vi "Handle.vi"(8 "error in (no error)":errorcluster, 11 "TelFocus in":refnum<class "TelFocus.lvclass">) -> (0 "error out":errorcluster, 3 "TelFocus out":refnum<class "TelFocus.lvclass">)   [LabVIEW 2018, in "TelFocus.lvclass"]
uses:
  TelFocus.lvclass
  TelFocus.lvclass/TelFocus.ctl
  Device/Device.lvclass/Device.ctl
  SecMirror/SecMirror.lvclass
  C:/Users/observer/Desktop/Sparc4GUI/Versao ZeroMQ/SPARC4_GUI -20240711_20240708/Device/Device.lvclass
  Server/Server.lvclass
  Comm/Stream/Stream.lvclass
  Device/Device.lvclass
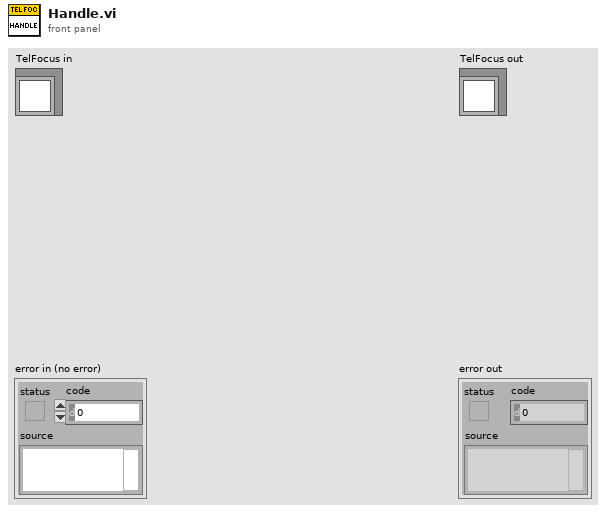
[diagram p1: front panel]
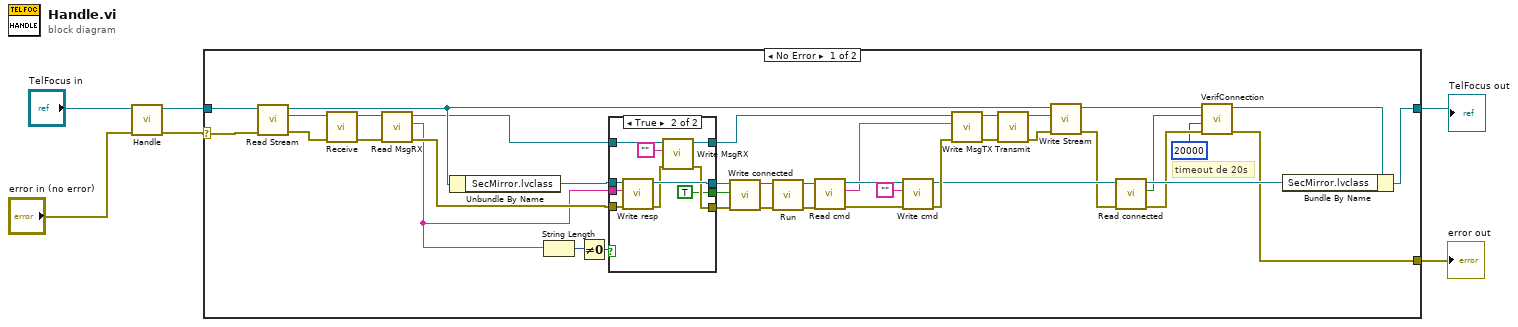
[diagram p0: block diagram]
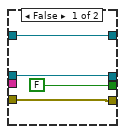
[diagram p2: hidden frame]
diagram:
  n1 = call-parent "Handle.vi"("error in (no error)"="error in (no error)", "Server in"="TelFocus in") -> ("error out"=w3:errorcluster, "Server out"=w4:refnum<class "TelFocus.lvclass">)  [unwired: 8 in]
  n2 = case shown="No Error" w3 {
    selector: w3 -> [w44 w62]
    tunnel: [w18 w62] -> w1
    tunnel: [w43 w61] -> w2
    tunnel: w4 -> [w35 w61]
    frame No Error {
      # "timeout de 20s"
      n3 = call-dynamic "Read Stream.vi"("error in (no error)"=w44, "Server in"=w35) -> ("error out"=w45:errorcluster, "Stream.lvclass"=w46:refnum<class "Stream.lvclass">, "Server out"=w37:refnum<class "TelFocus.lvclass">)  [unwired: 7 in]
      n4 = call-dynamic "Receive.vi"("error in (no error)"=w45, "Stream in"=w46) -> ("error out"=w42:errorcluster, "Stream out"=w41:refnum<class "Stream.lvclass">)  [unwired: 8 in]
      n5 = call-dynamic "Read MsgRX.vi"("error in (no error)"=w42, "Comm in"=w41) -> ("error out"=w15:errorcluster, "MsgRX"=w14:string, "Comm out"=w13:refnum<class "Stream.lvclass">)  [unwired: 7 in]
      n6 = Unbundle By Name(w37) -> ("SecMirror.lvclass"=w16:refnum<class "SecMirror.lvclass">)
      n7 = String Length(string=w14) -> (length=w29:i32)
      n8 = Not Equal To 0?(x=w29) -> (x != 0?=w28:bool)
      n9 = case shown="True" w28 {
        tunnel: [w49 w53] -> w9
        tunnel: [w50 w59] -> w10
        tunnel: w15 -> [w49 w58]
        tunnel: w16 -> [w50 w60]
        tunnel: w14 -> [_ w57]
        tunnel: w13 -> [w48 w56]
        tunnel: [w48 w55] -> w12
        tunnel: [FALSE TRUE] -> w11
        frame False {
        }
        frame True {
          n10 = call-dynamic "Write resp.vi"("error in (no error)"=w58, "resp"=w57, "Device in"=w60) -> ("error out"=w54:errorcluster, "Device out"=w59:refnum<class "SecMirror.lvclass">)  [unwired: 7 in]
          n11 = call-dynamic "Write MsgRX.vi"("error in (no error)"=w54, "MsgRX"="", "Comm in"=w56) -> ("error out"=w53:errorcluster, "Comm out"=w55:refnum<class "Stream.lvclass">)  [unwired: 7 in]
        }
      }
      n12 = call "Write connected.vi"("error in (no error)"=w9, "connected"=w11, "Device in"=w10) -> ("error out"=w7:errorcluster, "Device out"=w8:refnum<class "SecMirror.lvclass">)  [unwired: 7 in]
      n13 = call-dynamic "Run.vi"("error in (no error)"=w7, "SecMirror in"=w8) -> ("error out"=w26:errorcluster, "SecMirror out"=w27:refnum<class "SecMirror.lvclass">)  [unwired: 8 in]
      n14 = call-dynamic "Read cmd.vi"("error in (no error)"=w26, "Device in"=w27) -> ("error out"=w33:errorcluster, "cmd"=w31:string, "Device out"=w34:refnum<class "SecMirror.lvclass">)  [unwired: 7 in]
      n15 = call-dynamic "Write cmd.vi"("error in (no error)"=w33, "cmd"="", "Device in"=w34) -> ("error out"=w40:errorcluster, "Device out"=w25:refnum<class "SecMirror.lvclass">)  [unwired: 7 in]
      n16 = call-dynamic "Write MsgTX.vi"("error in (no error)"=w40, "MsgTX"=w31, "Comm in"=w12) -> ("error out"=w38:errorcluster, "Comm out"=w39:refnum<class "Stream.lvclass">)  [unwired: 7 in]
      n17 = call-dynamic "Transmit.vi"("error in (no error)"=w38, "Stream in"=w39) -> ("error out"=w36:errorcluster, "Stream out"=w30:refnum<class "Stream.lvclass">)  [unwired: 8 in]
      n18 = call-dynamic "Write Stream.vi"("error in (no error)"=w36, "Stream.lvclass"=w30, "Server in"=w37) -> ("error out"=w24:errorcluster, "Server out"=w23:refnum<class "TelFocus.lvclass">)  [unwired: 7 in]
      n19 = call "Read connected.vi"("error in (no error)"=w24, "Device in"=w25) -> ("error out"=w19:errorcluster, "connected"=w21:bool, "Device out"=w22:refnum<class "SecMirror.lvclass">)  [unwired: 7 in]
      n20 = call-dynamic "VerifConnection.vi"("error in (no error)"=w19, "timeout in ms (1000)"=u32 20000 ("period (ms)"), "device connected in"=w21, "Server in"=w23) -> ("error out"=w18:errorcluster, "Server out"=w20:refnum<class "TelFocus.lvclass">)  [unwired: 6 in]
      n21 = Bundle By Name(cluster=w20, "SecMirror.lvclass"=w22) -> (w43:refnum<class "TelFocus.lvclass">)
    }
    frame Error {
    }
  }
  "error out" <- w1
  "TelFocus out" <- w2
